vi "getLastFileName.vi"(9 "pattern":string="機台排程*.*", 11 "path":path=path "O:/mONITOR/REPORT") -> (2 "FileName":string)   [LabVIEW 2012]
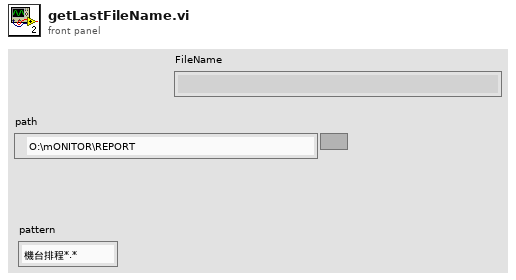
[diagram p1: front panel]
types:
  T1 = cluster{"date/time string":string, "date/time string":string}[]
  T2 = cluster{"date/time string":string, "date/time string":string}
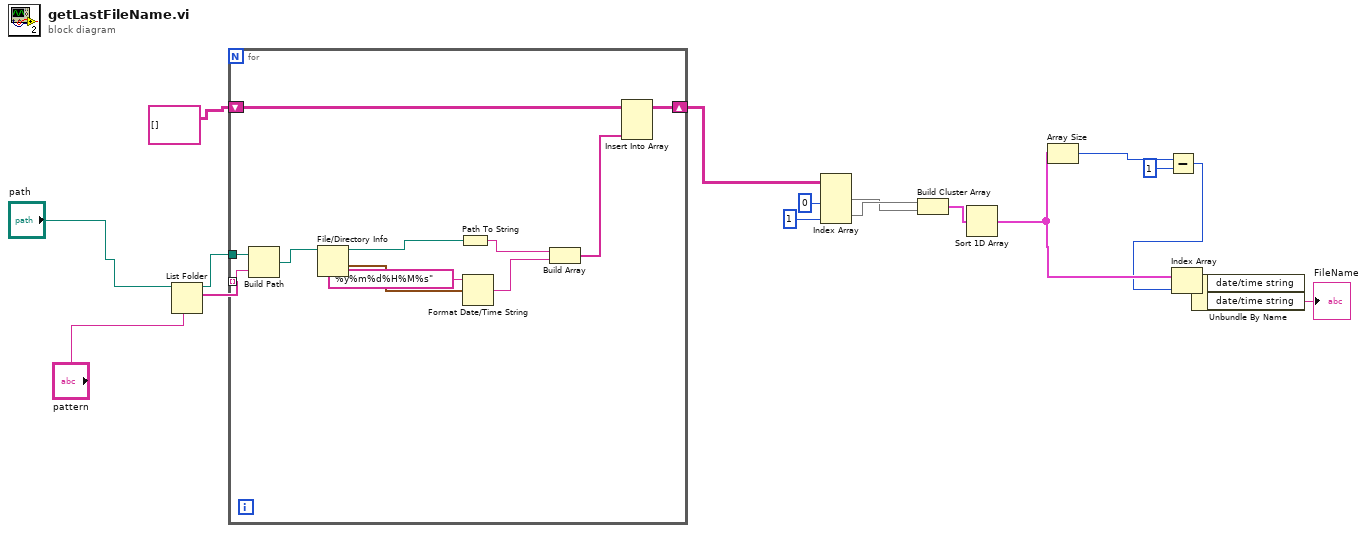
[diagram p0: block diagram]
diagram:
  n1 = List Folder(path="path", pattern="pattern") -> (path out=w16:path, filenames=w15:string[])  [unwired: 2 in, 2 out]
  n2 = for {
    tunnel: w16 -> [w28]
    tunnel: w15 -> [w27] mode=indexing
    shift-right: [w22] -> w13
    shift-left: string[][] [] ("array") -> [w21]
    n3 = Build Path(base path=w28, name or relative path=w27) -> (appended path=w26:path)
    n4 = File/Directory Info(path=w26) -> (path out=w25:path, last mod=w24:timestamp)  [unwired: 1 in, 5 out]
    n5 = Path To String(path=w25) -> (string=w20:string)
    n6 = Format Date/Time String(time format string (%c)="%y%m%d%H%M%s", seconds (now)=w24) -> (date/time string=w19:string)  [unwired: 1 in]
    n7 = Build Array(w20, w19) -> (w18:string[])
    n8 = Insert Into Array(array=w21, new element=w18) -> (w22:string[][])  [unwired: 2 in]
  }
  n9 = Index Array(array=w13, index (col) #1=0 ("disabled index (col)"), index (col) #2=1 ("index (col)")) -> (element #1=w8:string[], element #2=w9:string[])  [unwired: 2 in]
  n10 = Build Cluster Array(w9, w8) -> (w10:T1)
  n11 = Sort 1D Array(array=w10) -> (sorted array=w7:T1)
  n12 = Array Size(array=w7) -> (size(s)=w6:i32)
  n13 = Subtract(x=w6, y=1) -> (x-y=w4:i32)
  n14 = Index Array(array=w7, index=w4) -> (element=w3:T2)
  n15 = Unbundle By Name(w3) -> ("date/time string"=→"FileName":string)  [unwired: 1 out]
